vi "Core Action.vi"(8 "error in (no error)":errorcluster, 10 "SECS-II Class":refnum<class "SECS-II Class.lvclass">, 11 "16-Process Program Send in":refnum<class "16-Process Program Send.lvclass">) -> (0 "error out":errorcluster, 2 "SECS-II Class Out":refnum<class "SECS-II Class.lvclass">, 3 "16-Process Program Send out":refnum<class "16-Process Program Send.lvclass">)   [LabVIEW 2020, in "SECS Scenarios.lvlib" / "16-Process Program Send.lvclass"]
uses:
  16-Process Program Send.lvclass
  D:/Dropbox/SECS/SECS_GEM v1.1.0/Com/SECS Scenarios/Scenarios Class/Scenarios Class.lvclass
  SECS Communication/SECS-II Class/SECS-II Class.lvclass
  SECS Communication/S7 Message Class/S7 Message Class.lvclass
  D:/Dropbox/SECS/SECS_GEM v1.1.0/Com/SECS Communication/SECS-II Class/SECS-II Class.lvclass
  Scenarios Class/Reply State.ctl
  Scenarios Class/Scenarios Class.lvclass/Scenarios Class.ctl
  Scenarios Class/Write Reply State.vi
  Scenarios Class/Read HSMS Class.vi
  SECS Communication/HSMS Class/HSMS Class.lvclass
  Scenarios Class/Scenarios Class.lvclass
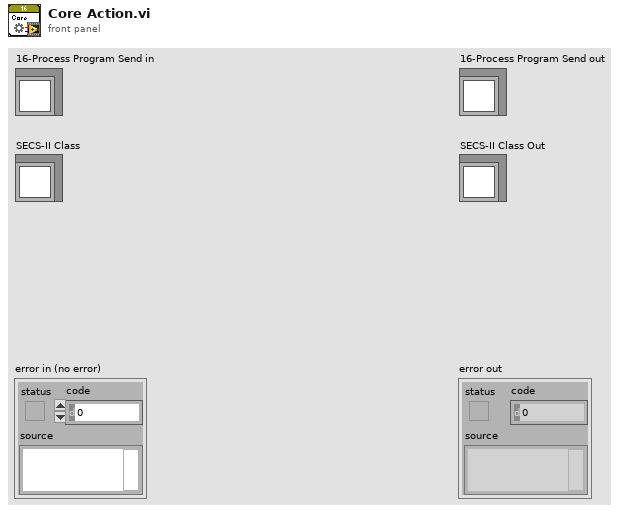
[diagram p1: front panel]
types:
  T1 = typedef "SECS Communication.lvlib/S7 Message Class.lvclass/S7F3.ctl" = cluster{"PPID":string, "PPBODY":u8[]}
  T2 = typedef "SECS Scenarios.lvlib/Scenarios Class.lvclass/Reply State.ctl" = enum16{"OK", "Illegal Data", "Unknown Stream", "Unknown Function", "Off-Line", "T3 Timeout", "Inner-Timeout"}
  T3 = typedef "SECS Communication.lvlib/S7 Message Class.lvclass/S7F4.ctl" = enum8{"Accepted", "Permission not granted", "length error", "matrix overflow", "PPID not found", "unsupported mode", "initiated for asynchronous completion", "storage limit error"}
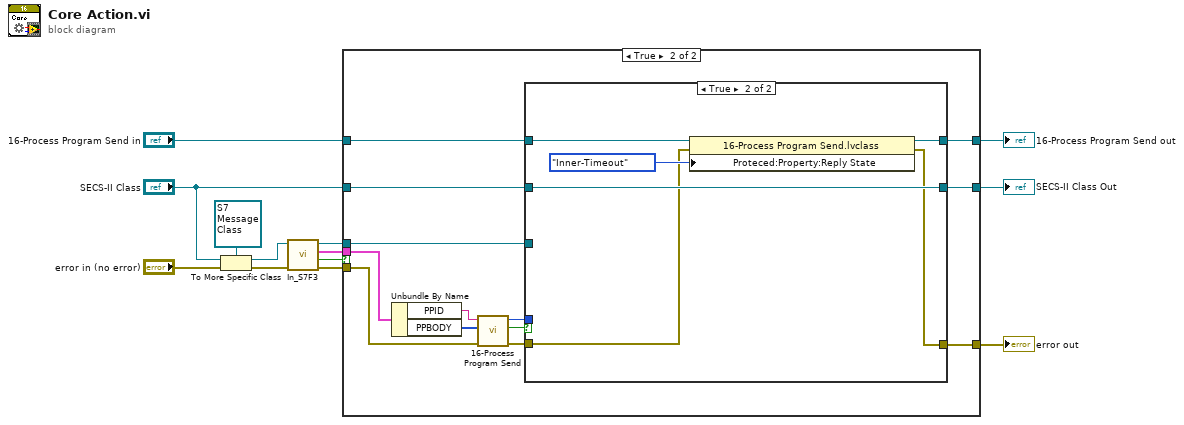
[diagram p0: block diagram]
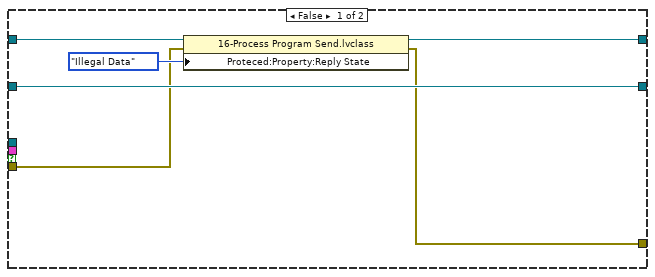
[diagram p2: hidden frame]
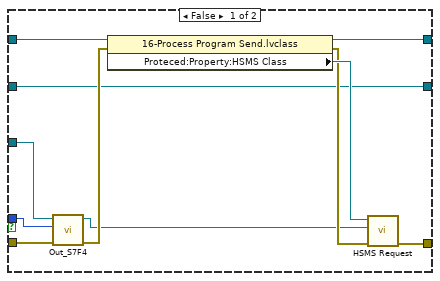
[diagram p3: hidden frame]
diagram:
  n1 = To More Specific Class(target class=refnum<class "S7 Message Class.lvclass"> refnum ("S7 Message Class in"), reference="SECS-II Class", error in="error in (no error)") -> (specific class reference=w11:refnum<class "S7 Message Class.lvclass">, error out=w12:errorcluster)
  n2 = call "In_S7F3.vi"("error in (no error)"=w12, "S7 Message Class in"=w11) -> ("error out"=w10:errorcluster, "OK?"=w1:bool, "S7F3"=w4:T1, "S7 Message Class out"=w9:refnum<class "S7 Message Class.lvclass">)  [unwired: 6 in]
  n3 = case shown="True" w1 {
    tunnel: w10 -> [w15 w32]
    tunnel: w9 -> [_ w28]
    tunnel: "16-Process Program Send in" -> [w19 w27]
    tunnel: [w16 w26] -> w6
    tunnel: [w14 w25] -> w5
    tunnel: w4 -> [_ w24]
    tunnel: "SECS-II Class" -> [w17 w21]
    tunnel: [w17 w20] -> w2
    frame False {
      n4 = property class="16-Process Program Send.lvclass"(reference=w19, error in=w15, "Proteced:Property:Reply State"=Reply_State."Illegal Data" ("Reply State")) -> (reference out=w16:refnum<class "16-Process Program Send.lvclass">, error out=w14:errorcluster)
    }
    frame True {
      n5 = Unbundle By Name(w24) -> ("PPID"=w22:string, "PPBODY"=w23:u8[])
      n6 = call "16-Process Program Send.vi"("error in (no error)"=w32, "PPBODY"=w23, "PPID"=w22) -> ("error out"=w31:errorcluster, "Timeout?"=w30:bool, "S7F4"=w29:T3)  [unwired: 6 in]
      n7 = case shown="True" w30 {
        tunnel: w27 -> [w43 w47]
        tunnel: w28 -> [w37 _]
        tunnel: [w40 w44] -> w25
        tunnel: [w39 w46] -> w26
        tunnel: w31 -> [w38 w45]
        tunnel: w29 -> [w34 _]
        tunnel: w21 -> [w33 w49]
        tunnel: [w33 w49] -> w20
        frame False {
          n8 = call "Out_S7F4.vi"("error in (no error)"=w38, "S7F4"=w34, "S7 Message Class in"=w37) -> ("error out"=w36:errorcluster, "S7 Message Class out"=w35:refnum<class "S7 Message Class.lvclass">)  [unwired: 7 in]
          n9 = property class="16-Process Program Send.lvclass"(reference=w43, error in=w36) -> (reference out=w39:refnum<class "16-Process Program Send.lvclass">, error out=w41:errorcluster, "Proteced:Property:HSMS Class"=w42:refnum<class "HSMS Class.lvclass">)
          n10 = call "HSMS Request.vi"("error in (no error)"=w41, "SECS-II Class In"=w35, "HSMS Class in"=w42) -> ("error out"=w40:errorcluster)  [unwired: 7 in, 1 out]
        }
        frame True {
          n11 = property class="16-Process Program Send.lvclass"(reference=w47, error in=w45, "Proteced:Property:Reply State"=Reply_State."Inner-Timeout" ("Reply State")) -> (reference out=w46:refnum<class "16-Process Program Send.lvclass">, error out=w44:errorcluster)
        }
      }
    }
  }
  "error out" <- w5
  "16-Process Program Send out" <- w6
  "SECS-II Class Out" <- w2
